vi "TCP2Foxconn_Main.vi"(8 "Error In":errorcluster, 11 "Name":string) -> (0 "Error Out":errorcluster)   [LabVIEW 2019, in "TCP2Foxconn.lvlib"]
uses:
  TCP2Foxconn.lvlib
  <vilib>/regexp/Match Regular Expression.xnode
  Queue/Queue.lvlib
  Data Error Notifier/Data and Error Notifier.lvlib
panel:
  out "Port":u16
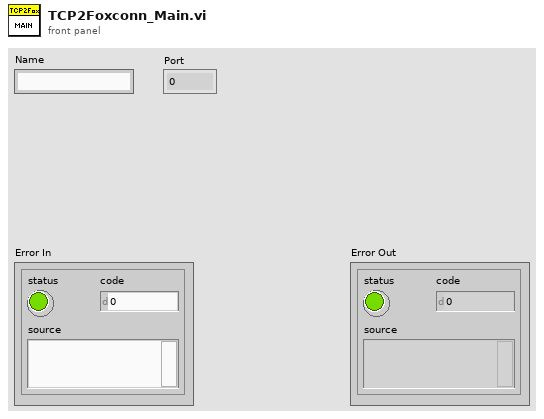
[diagram p1: front panel]
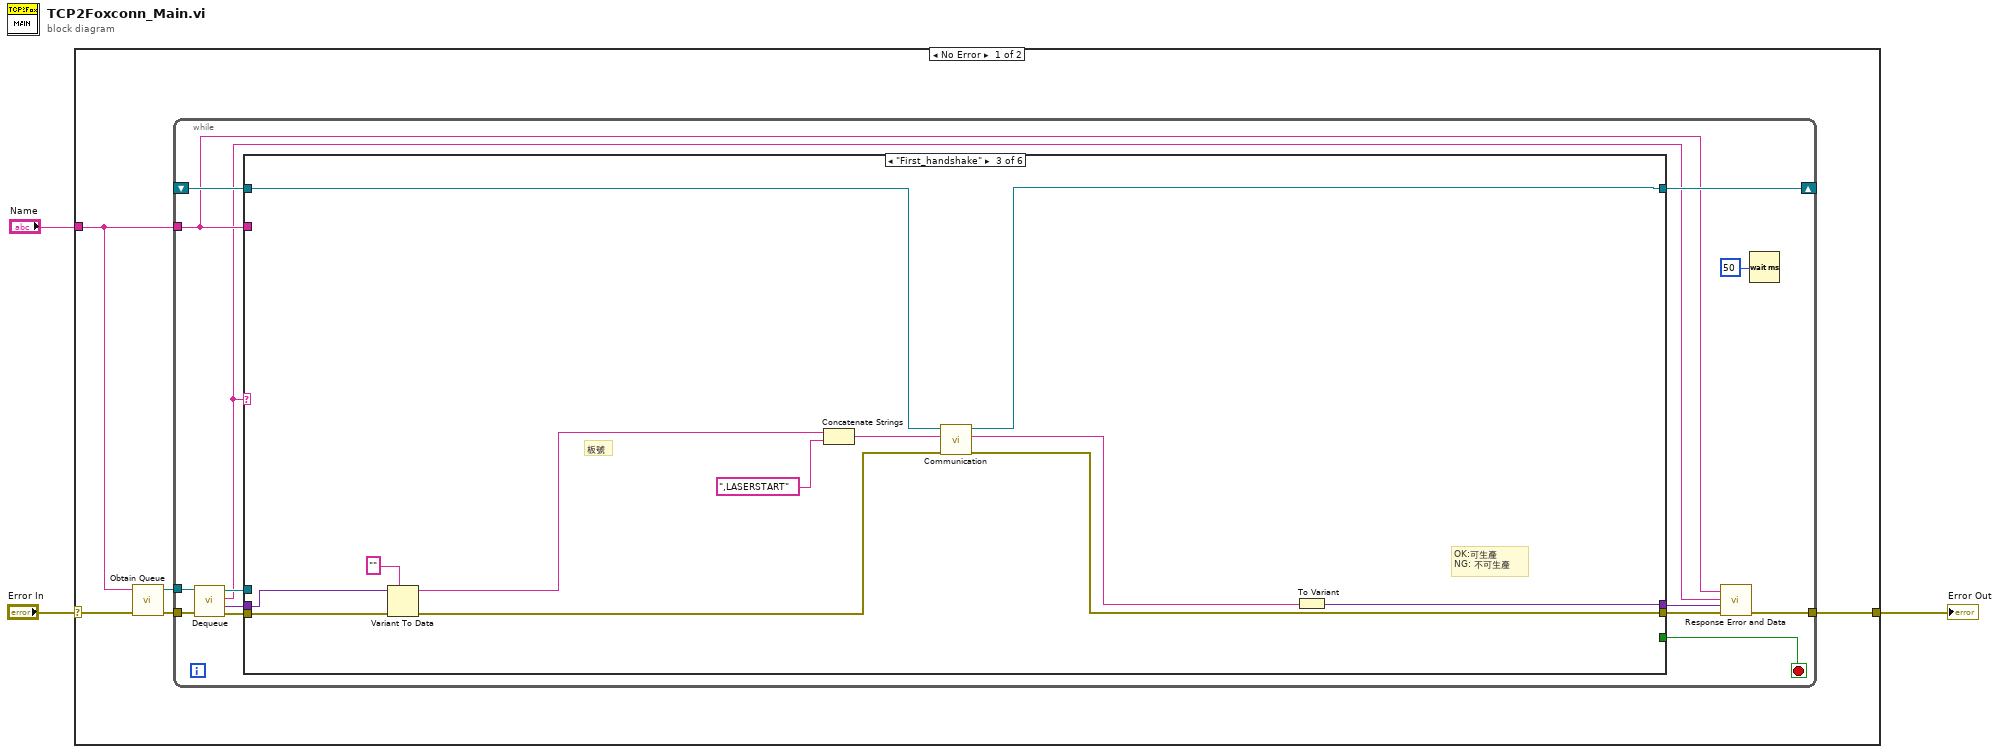
[diagram p0: block diagram]
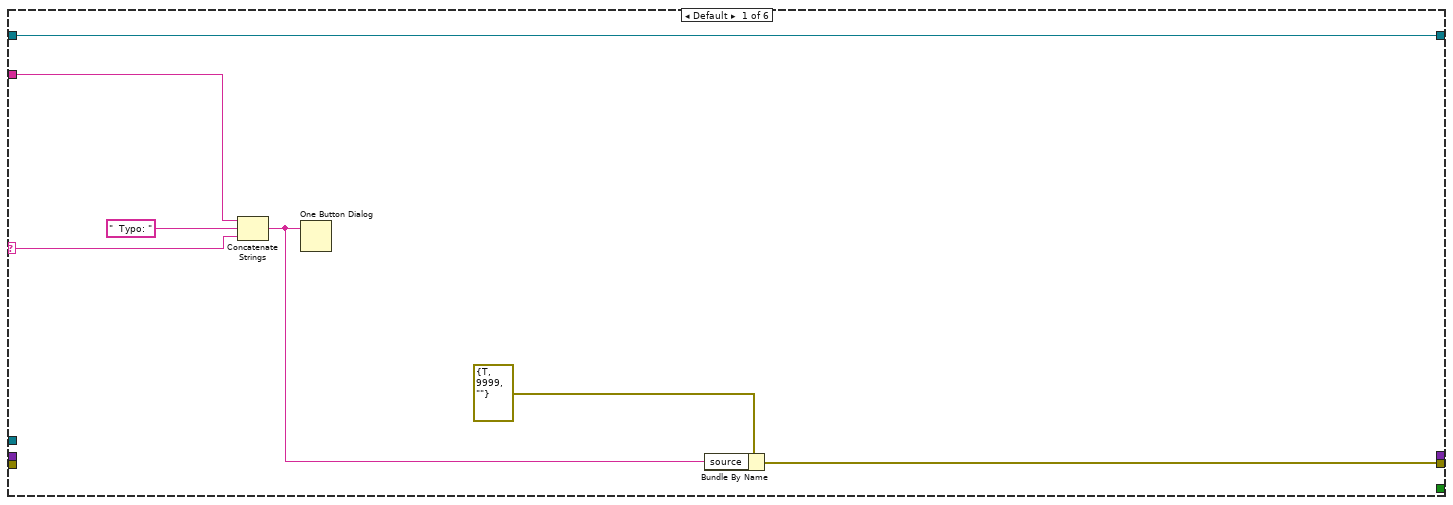
[diagram p2: hidden frame]
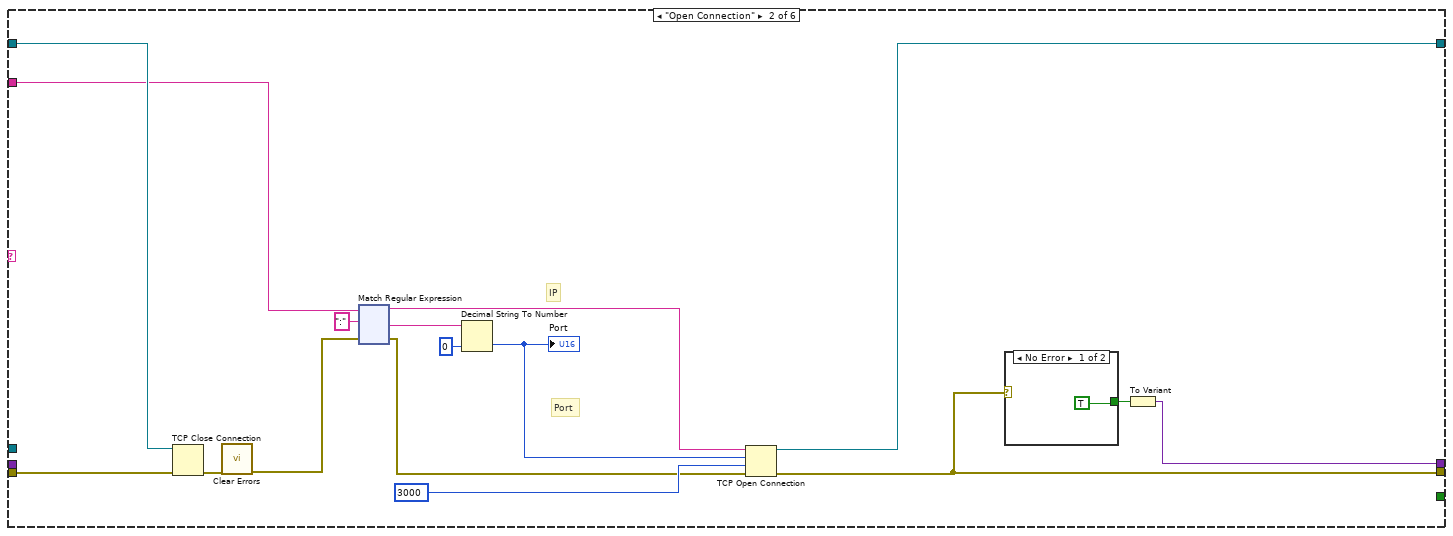
[diagram p3: hidden frame]
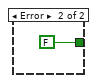
[diagram p4: hidden frame]
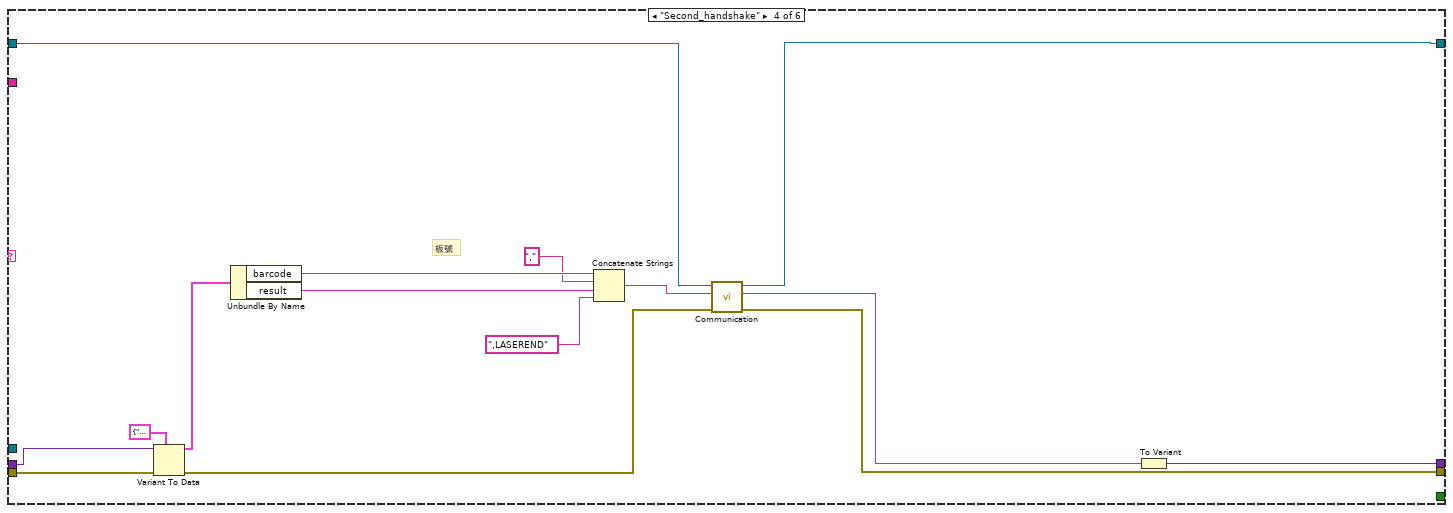
[diagram p5: hidden frame]
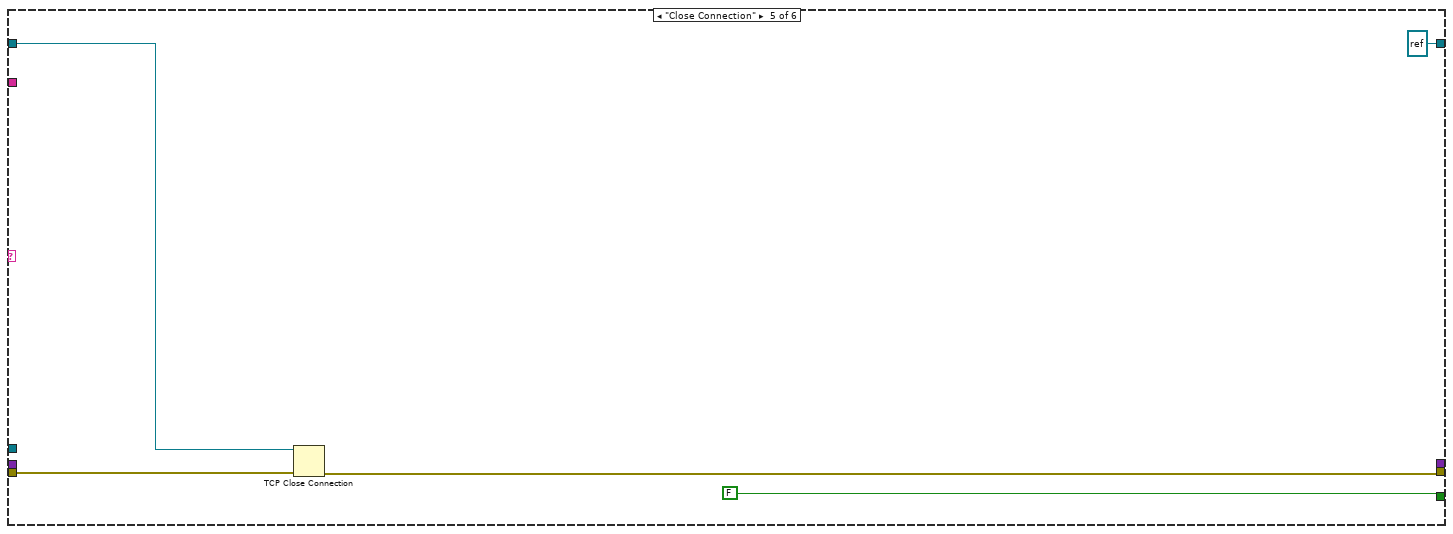
[diagram p6: hidden frame]
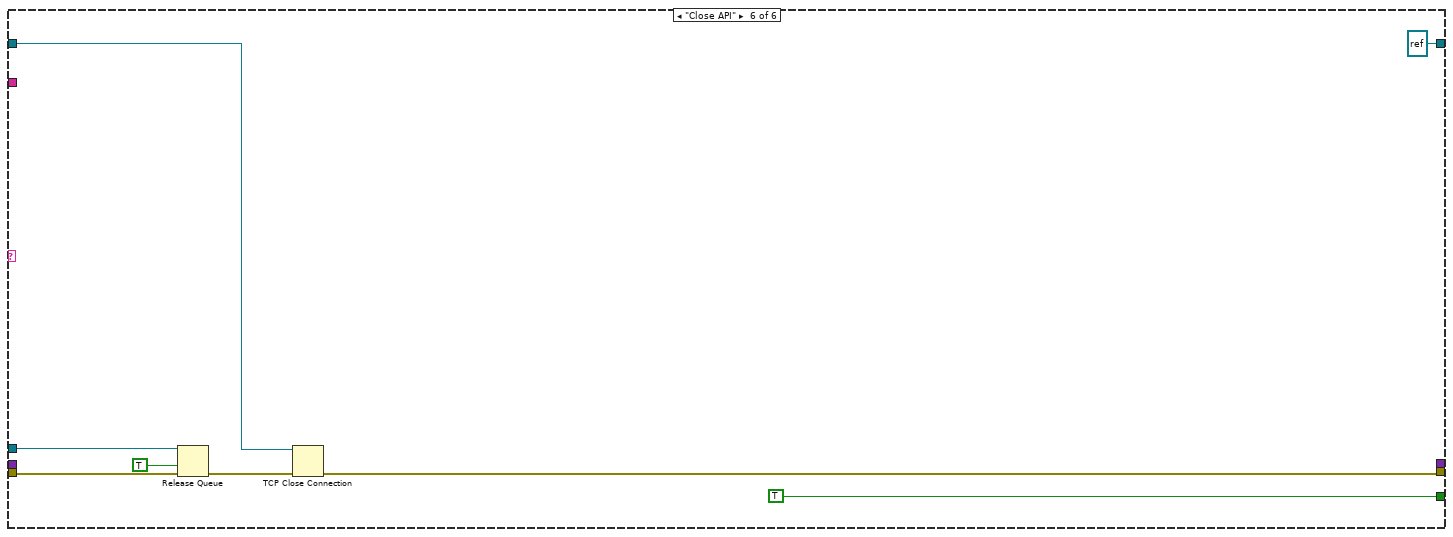
[diagram p7: hidden frame]
diagram:
  n1 = case shown="No Error" "Error In" {
    selector: "Error In" -> [w6 w202]
    tunnel: [w8 w202] -> w2
    tunnel: "Name" -> [w7 _]
    frame No Error {
      n2 = call "Obtain Queue.vi"("Error In"=w6, "Name"=w7) -> ("Error Out"=w4:errorcluster, "queue out"=w5:refnum<queue>)  [unwired: 8 in]
      n3 = while {
        tunnel: w7 -> [w14]
        tunnel: [w11] -> w8
        shift-right: [w21] -> _
        shift-left: _ -> [w22]
        tunnel: w5 -> [w19]
        tunnel: w4 -> [w18]
        stop <- w20 stop-if-true
        n4 = call "Dequeue.vi"("Error In"=w18, "queue in"=w19) -> ("Error Out"=w17:errorcluster, "Data"=w16:variant, "Message"=w13:string, "queue out"=w15:refnum<queue>)  [unwired: 6 in]
        n5 = case shown="\"First_handshake\"" w13 {
          selector: w13 -> [w27 _ _ _ _ _]
          tunnel: w17 -> [_ w45 w171 w186 w193 w200]
          tunnel: w14 -> [w29 w36 _ _ _ _]
          tunnel: w15 -> [_ _ _ _ _ w199]
          tunnel: [w24 w32 w164 w181 w191 w196] -> w12
          tunnel: w16 -> [_ _ w170 w185 _ _]
          tunnel: w22 -> [w23 w44 w173 w188 w192 w197]
          tunnel: [w23 w41 w172 w187 refnum<k5> refnum ("TCP Network Connection out") refnum<k5> refnum ("TCP Network Connection out")] -> w21
          tunnel: [_ _ _ _ FALSE TRUE] -> w20
          tunnel: [_ w30 w162 w174 _ _] -> w10
          frame Default {
            n6 = Concatenate Strings(w29, "  Typo: " ("string"), w27) -> (w25:string)
            n7 = One Button Dialog(message=w25) -> ()  [unwired: 1 in, 1 out]
            n8 = Bundle By Name(cluster=errorcluster {"status"=TRUE, "code"=9999, "source"=""} ("Error In"), "source"=w25) -> (w24:errorcluster)
          }
          frame "Open Connection" {
            # "Port"
            # "IP"
            n9 = TCP Close Connection(connection ID=w44, error in (no error)=w45) -> (error out=w43:errorcluster)  [unwired: 1 in, 1 out]
            n10 = call <vilib>:"Clear Errors.vi"("error in (no error)"=w43) -> ("error out"=w37:errorcluster)  [unwired: 5 in, 1 out]
            n11 = xnode "Match Regular Expression"("input string"=w36, "regular expression"=":", "error in"=w37) -> ("before match"=w34:string, "after match"=w39:string, "error out"=w35:errorcluster)  [unwired: 3 in, 2 out]
            n12 = Decimal String To Number(string=w39, default (0L)=u16 0 ("default (0 I32)")) -> (number=w33:u16)  [unwired: 1 in, 1 out]
            "Port" <- w33
            n13 = TCP Open Connection(address=w34, remote port or service name=w33, timeout ms (60000)=3000, error in (no error)=w35) -> (connection ID=w41:refnum<k5>, error out=w32:errorcluster)  [unwired: 1 in]
            n14 = case shown="No Error" w32 {
              tunnel: [TRUE FALSE] -> w31
              frame No Error {
              }
              frame Error {
              }
            }
            n15 = To Variant(anything=w31) -> (Variant=w30:variant)
          }
          frame "First_handshake" {
            # "OK:可生產\nNG: 不可生產"
            # "板號"
            n16 = Variant To Data(error in=w171, type="", Variant=w170) -> (data=w166:string, error out=w165:errorcluster)
            n17 = Concatenate Strings(w166, ",LASERSTART") -> (w167:string)
            n18 = call "Communication.vi"("Error In"=w165, "Command"=w167, "connection ID"=w173) -> ("Error Out"=w164:errorcluster, "Data out"=w163:string, "connection ID out"=w172:refnum<k5>)  [unwired: 6 in]
            n19 = To Variant(anything=w163) -> (Variant=w162:variant)
          }
          frame "Second_handshake" {
            # "板號"
            n20 = Variant To Data(error in=w186, type=cluster{"barcode":string, "result":string} {"barcode"="", "result"=""}, Variant=w185) -> (data=w179:cluster{"barcode":string, "result":string}, error out=w182:errorcluster)
            n21 = Unbundle By Name(w179) -> ("barcode"=w178:string, "result"=w176:string)
            n22 = Concatenate Strings(w178, "," ("string"), w176, ",LASEREND") -> (w183:string)
            n23 = call "Communication.vi"("Error In"=w182, "Command"=w183, "connection ID"=w188) -> ("Error Out"=w181:errorcluster, "Data out"=w175:string, "connection ID out"=w187:refnum<k5>)  [unwired: 6 in]
            n24 = To Variant(anything=w175) -> (Variant=w174:variant)
          }
          frame "Close Connection" {
            n25 = TCP Close Connection(connection ID=w192, error in (no error)=w193) -> (error out=w191:errorcluster)  [unwired: 1 in, 1 out]
          }
          frame "Close API" {
            n26 = Release Queue(queue=w199, force destroy? (F)=TRUE, error in (no error)=w200) -> (error out=w198:errorcluster)  [unwired: 2 out]
            n27 = TCP Close Connection(connection ID=w197, error in (no error)=w198) -> (error out=w196:errorcluster)  [unwired: 1 in, 1 out]
          }
        }
        n28 = call "Response Error and Data.vi"("error in (no error)"=w12, "Data In"=w10, "Message"=w13, "Name"=w14) -> ("error out"=w11:errorcluster)  [unwired: 5 in, 2 out]
        n29 = Wait (ms)(milliseconds to wait=u32 50) -> ()  [unwired: 1 out]
      }
    }
    frame Error {
    }
  }
  "Error Out" <- w2
